vi "rs3 Set All Advanced6.vi"(0 "Set Color Corr":bool=TRUE, 1 "Depth Presets":T2(ring), 2 "Color Presets":T1(ring), 7 "error in (no error)":errorcluster, 8 "device in":u64=370866768, 10 "ST_CensusEnable":cluster{"uDiameter":u32, "vDiameter":u32}={"uDiameter"=9, "vDiameter"=9}, 12 "ST_AE_Control":cluster{"meanIntensitySetpoint":u32}={"meanIntensitySetpoint"=400}, 16 "Depth Table":T3={"depthUnits, um"=1000, "depthClampMin"=0, "depthClampMax"=65535, "disparityMultiplier"=0, "disparityShift"=0}, 17 "ST RAU vector":T9={"minWest"=1, "minEast"=1, "minWEsum"=1, "minNorth"=1, "minSouth"=1, "minNSSum"=1, "uStrink"=1, "vShrink"=1}, 19 "ST Color Control":T8, 20 "depth control":T4={"plusIncrement"=10, "MinusDecrement"=10, "deepSeaMedianThreshold"=528, "scoreThreshA"=10, "scoreThreshB"=1023, "textureDifferenceThreshold"=0, "textureCountThreshold"=0, "deepSeaSecondPeakThreshold"=27, "deepSeaNeighborThreshold"=20, "IrAgreeThreshold"=70}, 21 "STColorCorrection":T11={"colorCorrection 1"=0.54785156, "colorCorrection 2"=0.32910156, "colorCorrection 3"=0.8222656, "colorCorrection 4"=0.109375, "colorCorrection 5"=-0.40527344, "colorCorrection 6"=-1.5253906, "colorCorrection 7"=0.95703125, "colorCorrection 8"=0.89160156, "colorCorrection 9"=0.7675781, "colorCorrection 10"=-0.4794922, "colorCorrection 11"=0.047851562, "colorCorrection 12"=-0.2705078}, 22 "HDAD":T12={"lambdaCensus"=26.0, "lambdaAD"=2100.0, "ignoreSAD"=0}, 23 "ST RSM":T10={"rsmBypass"=0, "diffThresh"=7.0, "sloRauDiffThresh"=3.0, "removeThresh"=33}, 24 "ST SLO Penalty":T5={"sloK1Penalty"=44, "sloK2Penalty"=502, "sloK1PenaltyMod1"=23, "sloK2PenaltyMod1"=237, "sloK1PenaltyMod2"=219, "sloK2PenaltyMod2"=113}, 25 "ST SLO Threshold":T6={"SLOdiffThresholdRed"=300, "SLODiffThresholdGreen"=300, "SLODiffThresholdBlue"=300}, 26 "ST Rau Threshold":T7={"rauDiffThresholdRed"=600, "rauDiffThresholdGreen"=600, "rauDiffThresholdBlue"=600}) -> (14 "Set advanced error":string, 18 "Dev out":u64=370866768, 27 "error out":errorcluster)   [LabVIEW 2019, in "libRealSense3.lvlib"]
doc: "The RealSense D4xx cameras are based on a stereo algorithm that has been accelerated as a fixed-function inside an ASIC. There are many parameters that affect the calculation of the depth. The basic task is to solve the correspondance problem - i.e. figure out which patches in the left image match up to those in the right image by doing a search along an epipolar line (x-axis). The x-axis difference for each object point is known as the disparity. \n\nIn general depth can be estimated for most points in the scene, but some points will have a very low confidence because 1. they are may be occluded (not seen by both imagers), or 2. have very little texture on them which will lead to an ambiquity (ex. when looking at a completely uniform white wall it, there are no best correspondances).\n\nThis VI allows you to set the many parameters that affect the algorith, as well as the color reproduction. \nNote that the color correction matrix will NOT have any effect on the depth calculations."
uses:
  libRealSense3.lvlib
panel:
  # "RS3 Set All Advanced 6"
  # "(C) 2017 Intel Corp.,  AGJ"
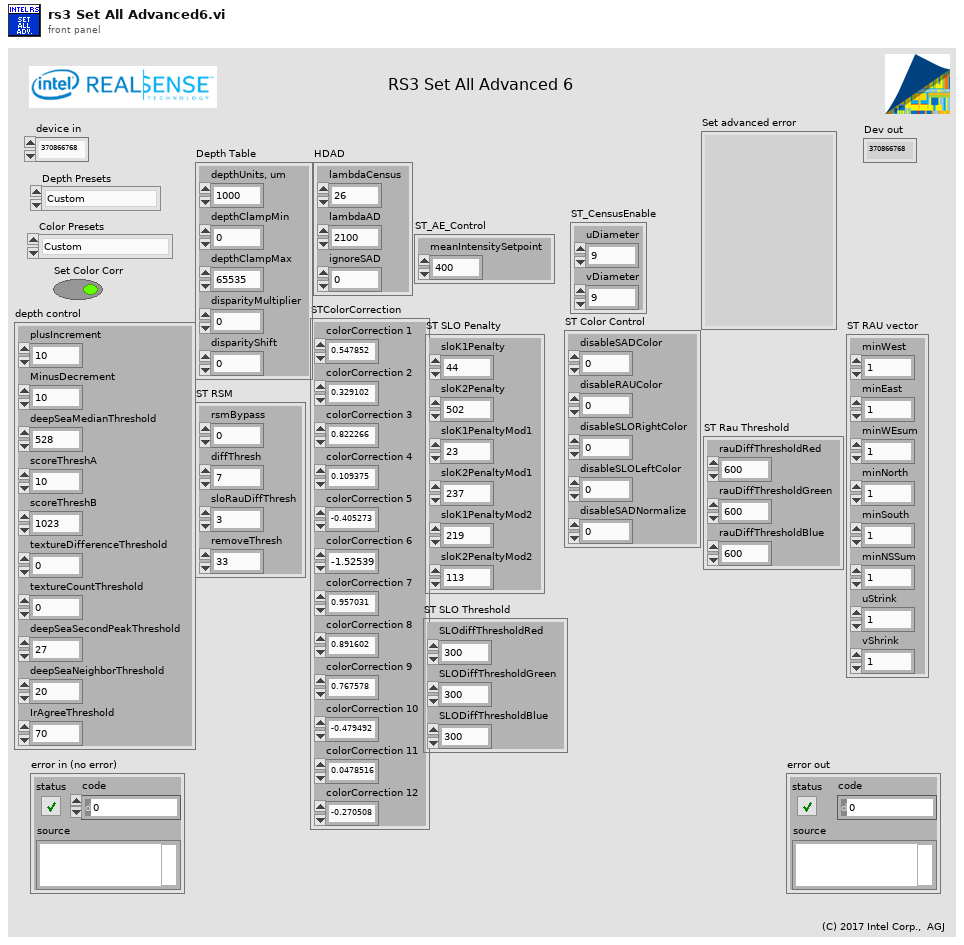
[diagram p1: front panel]
types:
  T1 = enum16{"Custom", "RS400 (DS5p)", "RS400 (DS5p) 2", "RS400 (DS5p) 3", "RS400 (DS5p) 4", "RS400 (DS5p) 5", "RS410 (DS5a)", "RS410 (DS5a) 2", "DS410 (DS5a) 3", "DS410 (DS5a) 4", "DS410+IR", "DS5LR", "DS5LR-2", "DS5LR no pattern", "RS410 Remove IR", "RS410 Remove IR 2", "DS5micro", "D435"}
  T2 = enum16{"Custom", "Original", "New Depth 1", "New Depth 2", "Depth Active 1", "Active 3D Scan", "Active Short A", "Active Short C", "Face", "Face2", "Best Box", "High Density", "Medium Density", "High Accuracy", "Hand", "Short Range", "Flat wall", "Load .JSON", "Load .JSON2"}
  T3 = cluster{"depthUnits, um":u32, "depthClampMin":u32, "depthClampMax":u32, "disparityMultiplier":u32, "disparityShift":u32}
  T4 = cluster{"plusIncrement":u32, "MinusDecrement":u32, "deepSeaMedianThreshold":u32, "scoreThreshA":u32, "scoreThreshB":u32, "textureDifferenceThreshold":u32, "textureCountThreshold":u32, "deepSeaSecondPeakThreshold":u32, "deepSeaNeighborThreshold":u32, "IrAgreeThreshold":u32}
  T5 = cluster{"sloK1Penalty":u32, "sloK2Penalty":u32, "sloK1PenaltyMod1":u32, "sloK2PenaltyMod1":u32, "sloK1PenaltyMod2":u32, "sloK2PenaltyMod2":u32}
  T6 = cluster{"SLOdiffThresholdRed":u32, "SLODiffThresholdGreen":u32, "SLODiffThresholdBlue":u32}
  T7 = cluster{"rauDiffThresholdRed":u32, "rauDiffThresholdGreen":u32, "rauDiffThresholdBlue":u32}
  T8 = cluster{"disableSADColor":u32, "disableRAUColor":u32, "disableSLORightColor":u32, "disableSLOLeftColor":u32, "disableSADNormalize":u32}
  T9 = cluster{"minWest":u32, "minEast":u32, "minWEsum":u32, "minNorth":u32, "minSouth":u32, "minNSSum":u32, "uStrink":u32, "vShrink":u32}
  T10 = cluster{"rsmBypass":u32, "diffThresh":sgl, "sloRauDiffThresh":sgl, "removeThresh":u32}
  T11 = cluster{"colorCorrection 1":sgl, "colorCorrection 2":sgl, "colorCorrection 3":sgl, "colorCorrection 4":sgl, "colorCorrection 5":sgl, "colorCorrection 6":sgl, "colorCorrection 7":sgl, "colorCorrection 8":sgl, "colorCorrection 9":sgl, "colorCorrection 10":sgl, "colorCorrection 11":sgl, "colorCorrection 12":sgl}
  T12 = cluster{"lambdaCensus":sgl, "lambdaAD":sgl, "ignoreSAD":u32}
  T13 = cluster{"rsmBypass (56)":u32, "diffThresh (57)":sgl, "sloRauDiffThresh(58)":sgl, "removeThresh(59)":u32}
  T14 = cluster{"depth control":cluster{"plusIncrement":u32, "MinusDecrement":u32, "deepSeaMedianThreshold":u32, "scoreThreshA":u32, "scoreThreshB":u32, "textureDifferenceThreshold":u32, "textureCountThreshold":u32, "deepSeaSecondPeakThreshold":u32, "deepSeaNeighborThreshold":u32, "IrAgreeThreshold":u32}, "STColorCorrection output":cluster{"colorCorrection 1":sgl, "colorCorrection 2":sgl, "colorCorrection 3":sgl, "colorCorrection 4":sgl, "colorCorrection 5":sgl, "colorCorrection 6":sgl, "colorCorrection 7":sgl, "colorCorrection 8":sgl, "colorCorrection 9":sgl, "colorCorrection 10":sgl, "colorCorrection 11":sgl, "colorCorrection 12":sgl}, "HDAD":cluster{"lambdaCensus":sgl, "lambdaAD":sgl, "ignoreSAD":u32}, "ST RSM":cluster{"rsmBypass":u32, "diffThresh":sgl, "sloRauDiffThresh":sgl, "removeThresh":u32}, "ST SLO Penalty":cluster{"sloK1Penalty":u32, "sloK2Penalty":u32, "sloK1PenaltyMod1":u32, "sloK2PenaltyMod1":u32, "sloK1PenaltyMod2":u32, "sloK2PenaltyMod2":u32}, "ST SLO Threshold":cluster{"SLOdiffThresholdRed":u32, "SLODiffThresholdGreen":u32, "SLODiffThresholdBlue":u32}, "ST Rau Threshold":cluster{"rauDiffThresholdRed":u32, "rauDiffThresholdGreen":u32, "rauDiffThresholdBlue":u32}, "ST Color Control":cluster{"disableSADColor":u32, "disableRAUColor":u32, "disableSLORightColor":u32, "disableSLOLeftColor":u32, "disableSADNormalize":u32}, "ST RAU vector":cluster{"minWest":u32, "minEast":u32, "minWEsum":u32, "minNorth":u32, "minSouth":u32, "minNSSum":u32, "uStrink":u32, "vShrink":u32}, "Depth Table":cluster{"depthUnits, um":u32, "depthClampMin":u32, "depthClampMax":u32, "disparityMultiplier":u32, "disparityShift":u32}, "ST_AE_Control":cluster{"meanIntensitySetpoint":u32}, "ST_CensusEnable":cluster{"uDiameter":u32, "vDiameter":u32}}
  T15 = cluster{"depthUnits, um":u32, "depthClampMin":u32, "depthClampMax":u32, "disparityMultiplier":u32, "disparityShift(0-127)":u32}
  T16 = cluster{"minWest (60)":u32, "minEast (61)":u32, "minWEsum (62)":u32, "minNorth (63)":u32, "minSouth (64)":u32, "minNSSum(65)":u32, "uStrink (66)":u32, "vShrink (67)":u32}
  T17 = cluster{"rauDiffThreshRed(73)":u32, "rauDiffThreshGreen(74)":u32, "rauDiffThreshBlue(75)":u32}
  T18 = cluster{"sloK1Penalty (79)":u32, "sloK2Penalty (80)":u32, "sloK1PenaltyMod1(81)":u32, "sloK2PenaltyMod1(82)":u32, "sloK1PenaltyMod2(83)":u32, "sloK2PenaltyMod2(84)":u32}
  T19 = cluster{"SLOdiffThreshRed(76)":u32, "SLODiffThreshGreen(77)":u32, "SLODiffThreshBlue(78)":u32}
  T20 = cluster{"disableSADColor(68)":u32, "disableRAUColor(69)":u32, "disableSLORightColor(70)":u32, "disableSLOLeftColor(71)":u32, "disableSADNormalize(72)":u32}
  T21 = cluster{"plusIncrement (47)":u32, "MinusDecrement (46)":u32, "deepSeaMedianThreshold (48)":u32, "scoreThreshA(49)":u32, "scoreThreshB (50)":u32, "textureDifferenceThreshold (52)":u32, "textureCountThreshold (51)":u32, "deepSea2ndPeakThresh.(53)":u32, "deepSeaNeighborThresh.(54)":u32, "LRAgreeThreshold (55)":u32}
  T22 = cluster{"plusIncrement (47)":u32, "MinusDecrement (46)":u32, "deepSeaMedianThreshold (48)":u32, "scoreThreshA(49)":u32, "scoreThreshB (50)":u32, "textureDifferenceThreshold (52)":u32, "textureCountThreshold (51)":u32, "deepSea2ndPeakThresh.(53)":u32, "deepSeaNeighborThresh.(54)":u32, "IrAgreeThreshold (55)":u32}
  T23 = cluster{"DS5p- 1":sgl, "colorCorrection 2":sgl, "colorCorrection 3":sgl, "colorCorrection 4":sgl, "colorCorrection 5":sgl, "colorCorrection 6":sgl, "colorCorrection 7":sgl, "colorCorrection 8":sgl, "colorCorrection 9":sgl, "colorCorrection 10":sgl, "colorCorrection 11":sgl, "colorCorrection 12":sgl}
  T24 = cluster{"Color 0":dbl, "Color 1":dbl, "Color 2":dbl, "Color 3":dbl, "Color 4":dbl, "Color 5":dbl, "Color 6":dbl, "Color 7":dbl, "Color 8":dbl, "Color 9":dbl, "Color 10":dbl, "Color 11":dbl}
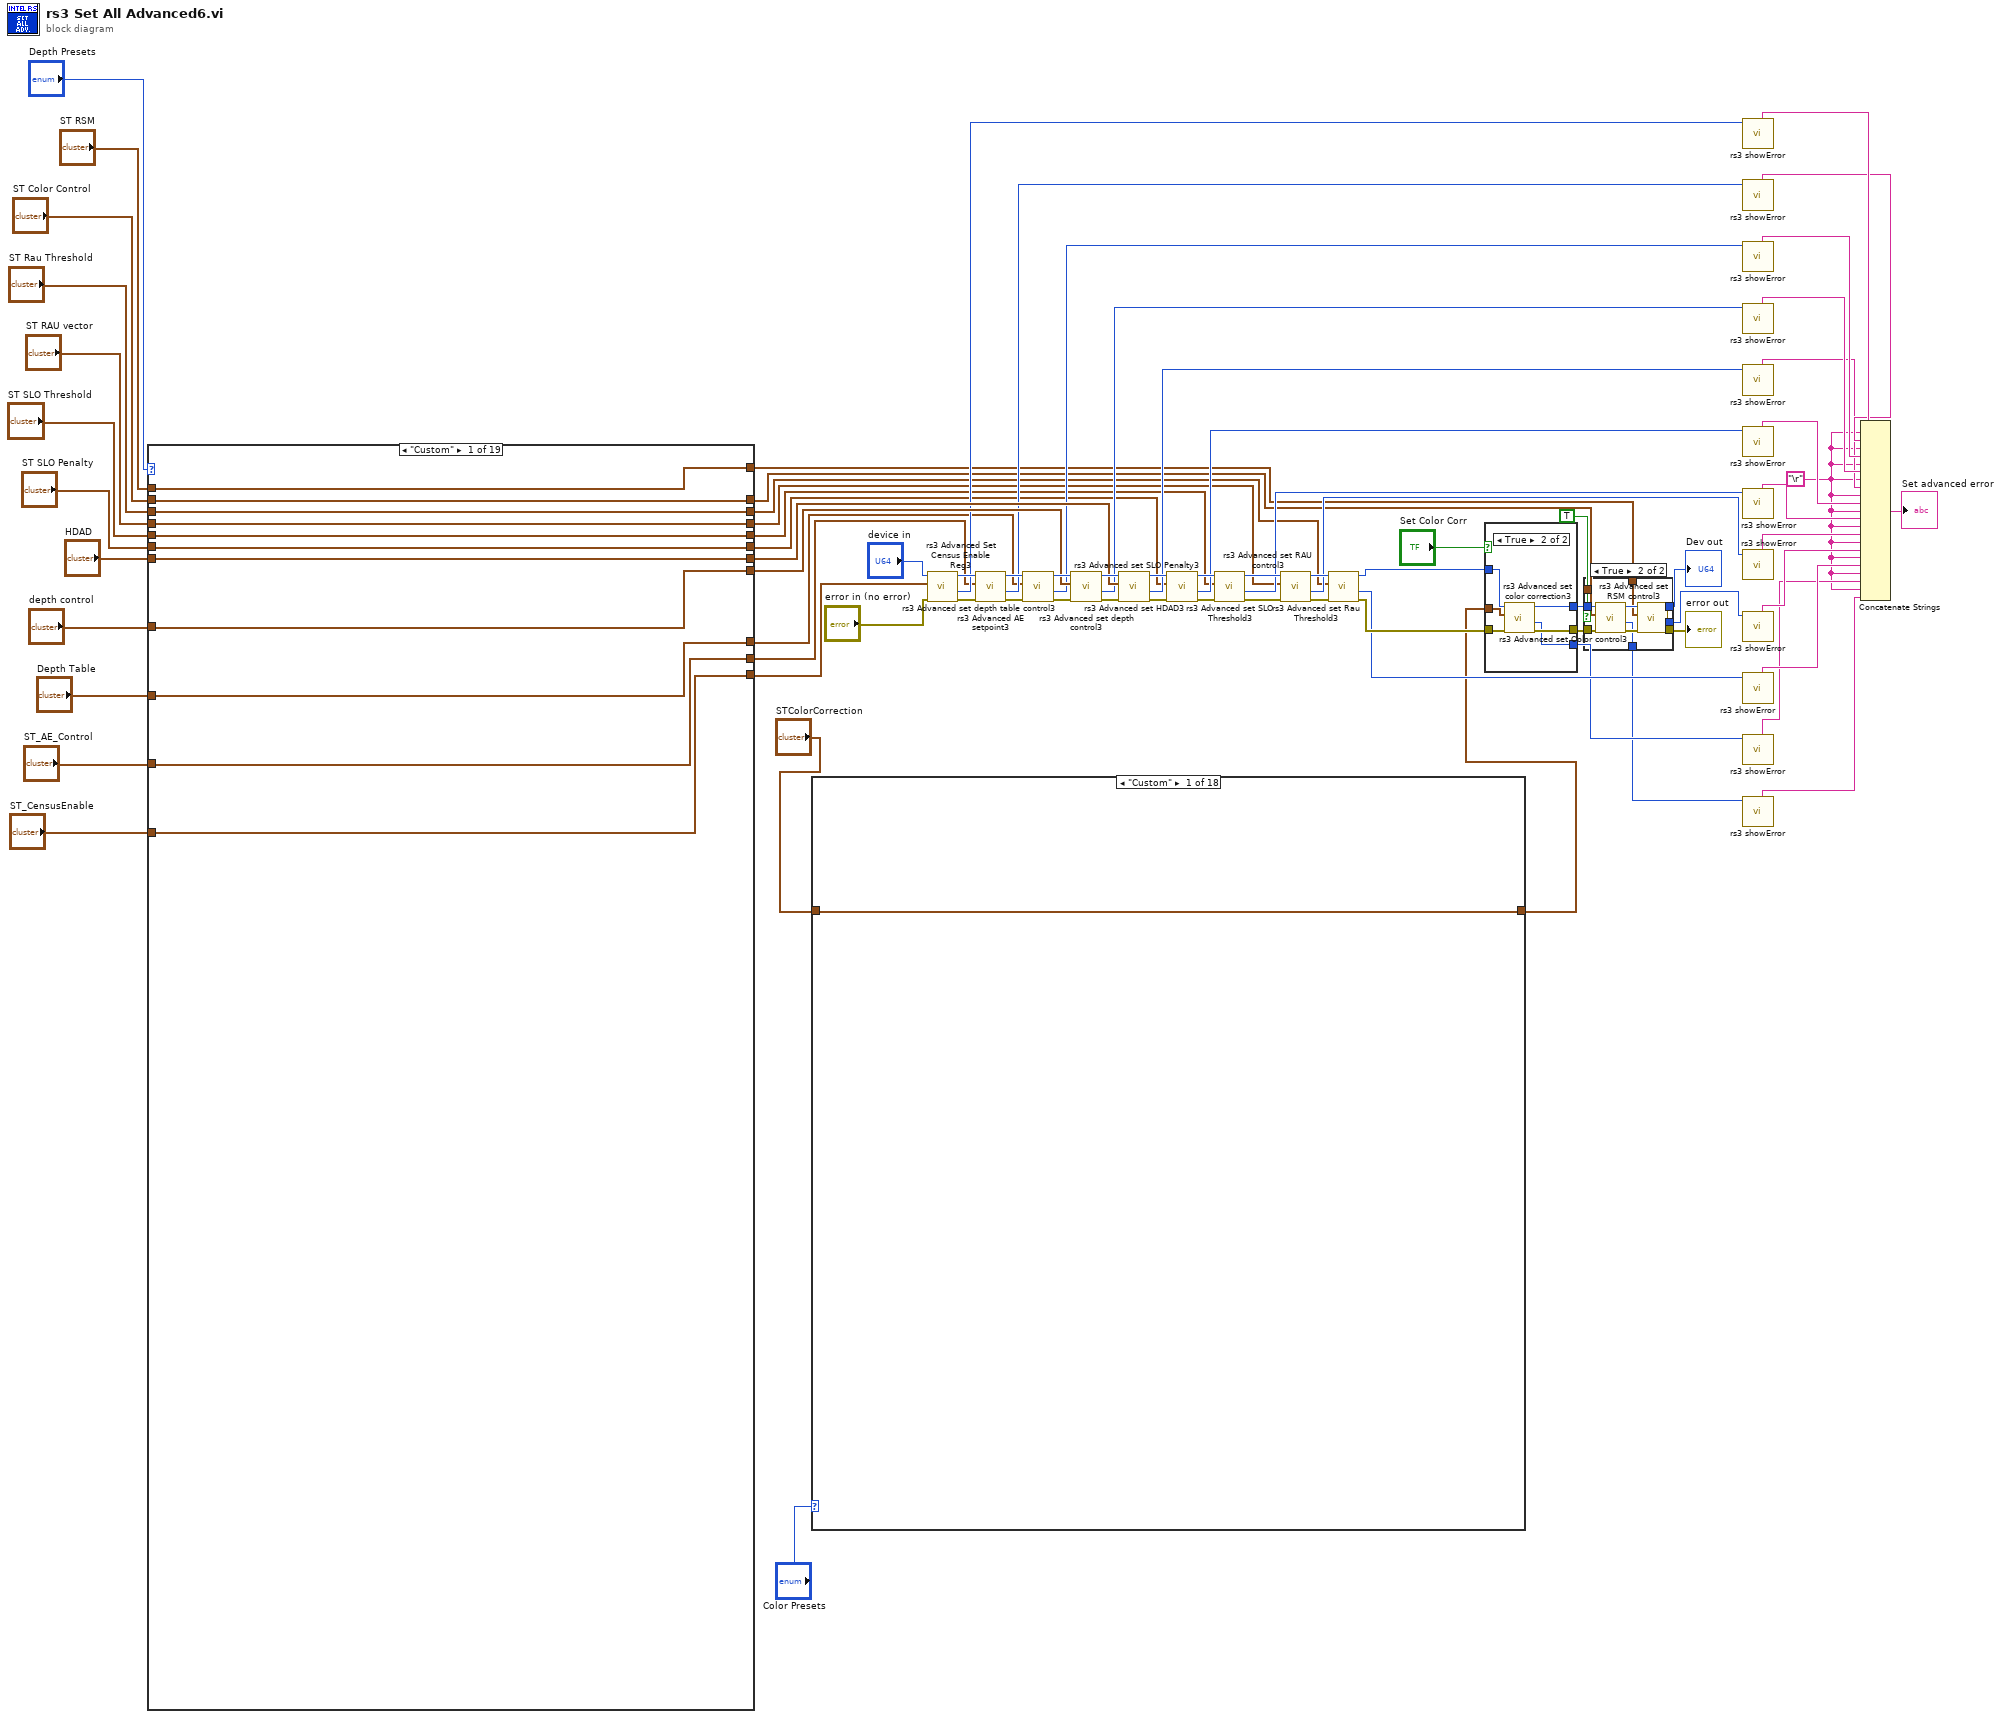
[diagram p0: block diagram]
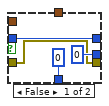
[diagram p2: hidden frame]
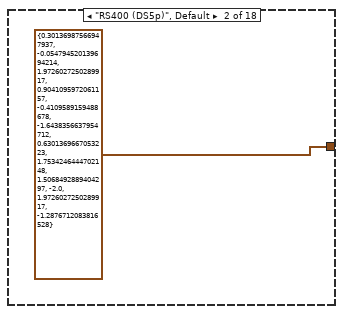
[diagram p3: hidden frame]
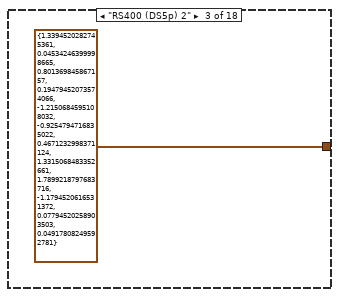
[diagram p4: hidden frame]
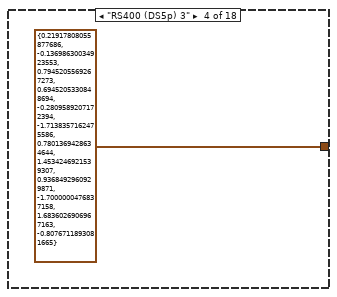
[diagram p5: hidden frame]
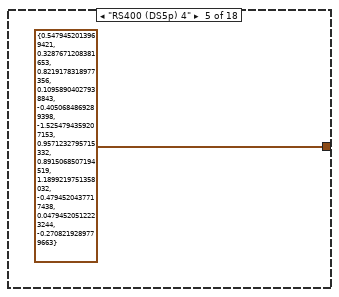
[diagram p6: hidden frame]
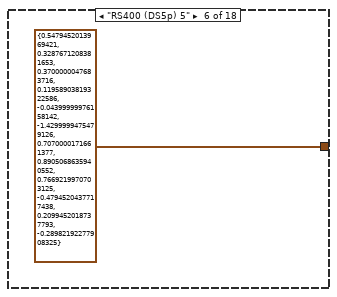
[diagram p7: hidden frame]
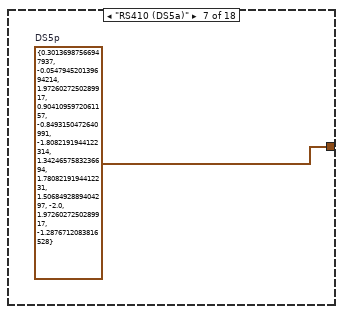
[diagram p8: hidden frame]
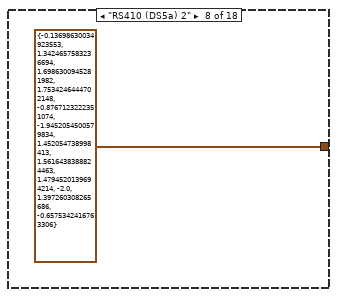
[diagram p9: hidden frame]
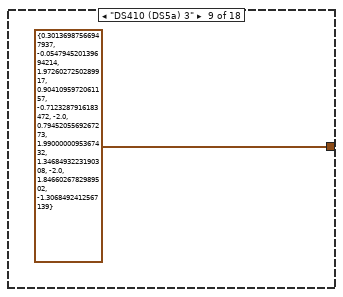
[diagram p10: hidden frame]
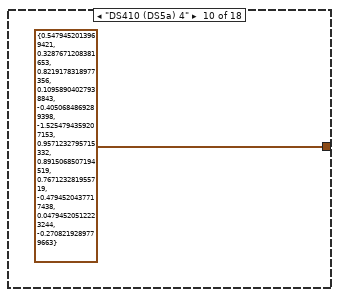
[diagram p11: hidden frame]
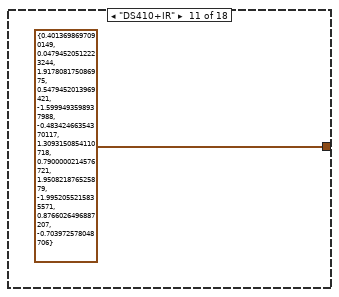
[diagram p12: hidden frame]
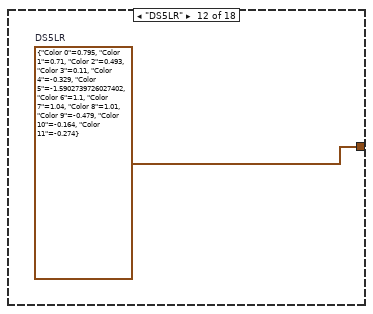
[diagram p13: hidden frame]
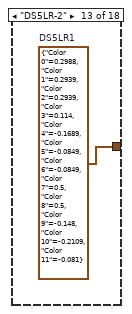
[diagram p14: hidden frame]
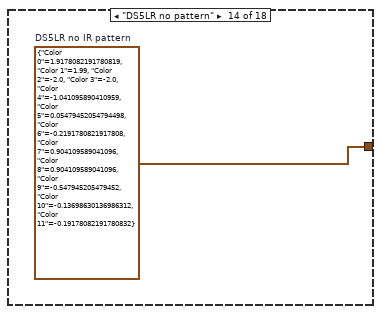
[diagram p15: hidden frame]
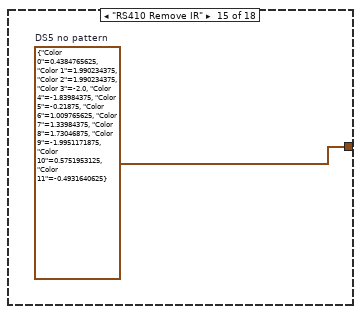
[diagram p16: hidden frame]
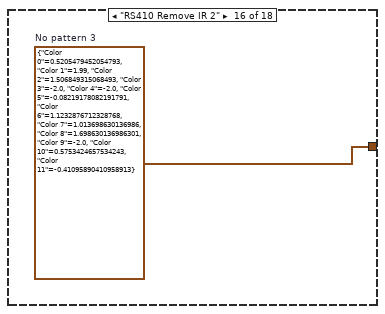
[diagram p17: hidden frame]
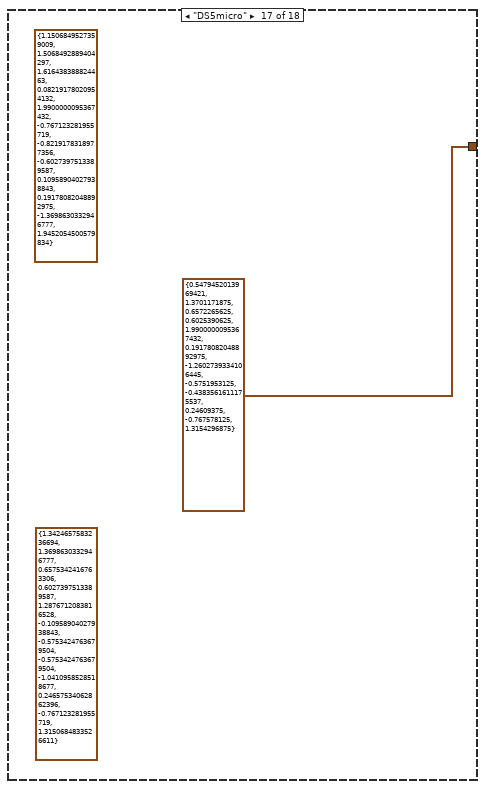
[diagram p18: hidden frame]
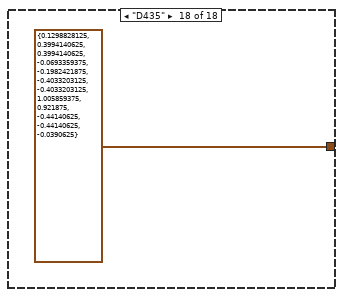
[diagram p19: hidden frame]
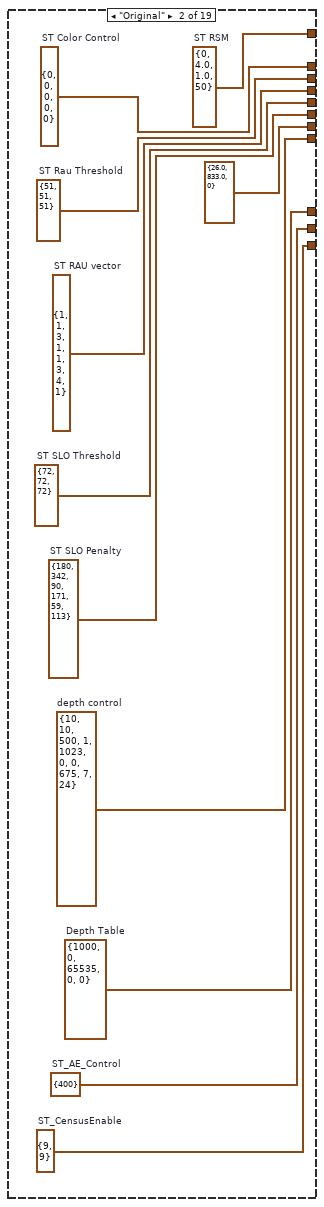
[diagram p20: hidden frame]
diagram:
  w24 = "\r"
  n1 = case shown="\"Custom\"" "Depth Presets" {
    tunnel: [w89 w99 w111 w122 w133 w137 w148 w159 w175 w185 w196 w203 w216 w228 w240 w252 w264 w279 w293] -> w51
    tunnel: [w83 w98 w110 w121 w132 T13 {"rsmBypass (56)"=0, "diffThresh (57)"=1.0367311, "sloRauDiffThresh(58)"=151.0, "removeThresh(59)"=1} ("ST RSM 2") w155 w166 w177 w182 w193 w208 w221 w233 w245 w257 w269 w281 w295] -> w13
    tunnel: [w84 w93 w109 w120 w131 w144 w154 w165 w176 w183 w194 w210 w223 w235 w247 w259 w271 w278 w292] -> w15
    tunnel: [w85 w94 w108 w119 w130 w143 w153 w164 w173 w184 w195 w206 w219 w231 w243 w255 w267 w282 w296] -> w16
    tunnel: [w82 w97 w107 w118 w129 w142 w152 w163 w172 w186 w197 w202 w215 w227 w239 w251 w263 w285 w299] -> w11
    tunnel: [w86 w96 w106 w117 w128 w141 w151 w162 w170 w187 w198 w201 w214 w226 w238 w250 w262 w284 w298] -> w18
    tunnel: [w87 w95 w105 w116 w127 w140 w150 w161 w174 w188 w199 w200 w213 w225 w237 w249 w261 w283 w297] -> w21
    tunnel: [w88 T12 {"lambdaCensus"=26.0, "lambdaAD"=833.0, "ignoreSAD"=0} ("HDAD 2") T12 {"lambdaCensus"=126.0, "lambdaAD"=800.0, "ignoreSAD"=0} ("HDAD 2") T12 {"lambdaCensus"=200.0, "lambdaAD"=1900.0, "ignoreSAD"=0} ("HDAD 2") T12 {"lambdaCensus"=216.0, "lambdaAD"=1400.0, "ignoreSAD"=0} ("HDAD 2") T12 {"lambdaCensus"=26.0, "lambdaAD"=833.0, "ignoreSAD"=0} ("HDAD 2") T12 {"lambdaCensus"=100.0, "lambdaAD"=1600.0, "ignoreSAD"=0} ("HDAD 2") w160 w171 T12 {"lambdaCensus"=26.0, "lambdaAD"=2100.0, "ignoreSAD"=0} ("HDAD*") T12 {"lambdaCensus"=15.0, "lambdaAD"=618.0, "ignoreSAD"=0} ("HDAD*") w209 w222 w234 w246 w258 w270 w280 w294] -> w49
    tunnel: [w80 w90 w101 w112 w123 w134 w145 w157 w167 w178 w189 w204 w217 w229 w241 w253 w265 w272 w288] -> w7
    tunnel: [w81 w91 w102 w113 w124 w135 w146 w156 w168 w179 w190 w205 w218 w230 w242 w254 w266 w273 w287] -> w9
    tunnel: [w79 w92 w103 w114 w125 w136 w147 w158 w169 w180 w191 w207 w220 w232 w244 w256 w268 w274 w286] -> w5
    tunnel: "depth control" -> [w89 _ _ _ _ _ _ _ _ _ _ _ _ _ _ _ _ _ _]
    tunnel: "HDAD" -> [w88 _ _ _ _ _ _ _ _ _ _ _ _ _ _ _ _ _ _]
    tunnel: "ST SLO Penalty" -> [w87 _ _ _ _ _ _ _ _ _ _ _ _ _ _ _ _ _ _]
    tunnel: "ST SLO Threshold" -> [w86 _ _ _ _ _ _ _ _ _ _ _ _ _ _ _ _ _ _]
    tunnel: "ST RAU vector" -> [w84 _ _ _ _ _ _ _ _ _ _ _ _ _ _ _ _ _ _]
    tunnel: "ST Rau Threshold" -> [w85 _ _ _ _ _ _ _ _ _ _ _ _ _ _ _ _ _ _]
    tunnel: "ST RSM" -> [w83 _ _ _ _ _ _ _ _ _ _ _ _ _ _ _ _ _ _]
    tunnel: "ST Color Control" -> [w82 _ _ _ _ _ _ _ _ _ _ _ _ _ _ _ _ _ _]
    tunnel: "ST_CensusEnable" -> [w81 _ _ _ _ _ _ _ _ _ _ _ _ _ _ _ _ _ _]
    tunnel: "ST_AE_Control" -> [w80 _ _ _ _ _ _ _ _ _ _ _ _ _ _ _ _ _ _]
    tunnel: "Depth Table" -> [w79 _ _ _ _ _ _ _ _ _ _ _ _ _ _ _ _ _ _]
    frame "Custom" {
    }
    frame "Original" {
      w91 = cluster{"uDiameter":u32, "vDiameter":u32} {"uDiameter"=9, "vDiameter"=9}  # ST_CensusEnable
      w92 = T15 {"depthUnits, um"=1000, "depthClampMin"=0, "depthClampMax"=65535, "disparityMultiplier"=0, "disparityShift(0-127)"=0}  # Depth Table
      w90 = cluster{"meanIntensitySetpoint":u32} {"meanIntensitySetpoint"=400}  # ST_AE_Control
      w93 = T16 {"minWest (60)"=1, "minEast (61)"=1, "minWEsum (62)"=3, "minNorth (63)"=1, "minSouth (64)"=1, "minNSSum(65)"=3, "uStrink (66)"=4, "vShrink (67)"=1}  # ST RAU vector
      w94 = T17 {"rauDiffThreshRed(73)"=51, "rauDiffThreshGreen(74)"=51, "rauDiffThreshBlue(75)"=51}  # ST Rau Threshold
      w95 = T18 {"sloK1Penalty (79)"=180, "sloK2Penalty (80)"=342, "sloK1PenaltyMod1(81)"=90, "sloK2PenaltyMod1(82)"=171, "sloK1PenaltyMod2(83)"=59, "sloK2PenaltyMod2(84)"=113}  # ST SLO Penalty
      w96 = T19 {"SLOdiffThreshRed(76)"=72, "SLODiffThreshGreen(77)"=72, "SLODiffThreshBlue(78)"=72}  # ST SLO Threshold
      w97 = T20 {"disableSADColor(68)"=0, "disableRAUColor(69)"=0, "disableSLORightColor(70)"=0, "disableSLOLeftColor(71)"=0, "disableSADNormalize(72)"=0}  # ST Color Control
      w98 = T13 {"rsmBypass (56)"=0, "diffThresh (57)"=4.0, "sloRauDiffThresh(58)"=1.0, "removeThresh(59)"=50}  # ST RSM
      w99 = T21 {"plusIncrement (47)"=10, "MinusDecrement (46)"=10, "deepSeaMedianThreshold (48)"=500, "scoreThreshA(49)"=1, "scoreThreshB (50)"=1023, "textureDifferenceThreshold (52)"=0, "textureCountThreshold (51)"=0, "deepSea2ndPeakThresh.(53)"=675, "deepSeaNeighborThresh.(54)"=7, "LRAgreeThreshold (55)"=24}  # depth control
    }
    frame "New Depth 1", Default {
      w102 = cluster{"uDiameter":u32, "vDiameter":u32} {"uDiameter"=9, "vDiameter"=9}  # ST_CensusEnable
      w103 = T15 {"depthUnits, um"=1000, "depthClampMin"=0, "depthClampMax"=65535, "disparityMultiplier"=0, "disparityShift(0-127)"=0}  # Depth Table
      w101 = cluster{"meanIntensitySetpoint":u32} {"meanIntensitySetpoint"=400}  # ST_AE_Control
      w105 = T18 {"sloK1Penalty (79)"=42, "sloK2Penalty (80)"=191, "sloK1PenaltyMod1(81)"=84, "sloK2PenaltyMod1(82)"=4, "sloK1PenaltyMod2(83)"=59, "sloK2PenaltyMod2(84)"=4}  # ST SLO Penalty 2
      w106 = T19 {"SLOdiffThreshRed(76)"=43, "SLODiffThreshGreen(77)"=83, "SLODiffThreshBlue(78)"=72}  # ST SLO Threshold 2
      w107 = T20 {"disableSADColor(68)"=0, "disableRAUColor(69)"=0, "disableSLORightColor(70)"=0, "disableSLOLeftColor(71)"=0, "disableSADNormalize(72)"=0}  # ST Color Control 2
      w108 = T17 {"rauDiffThreshRed(73)"=1, "rauDiffThreshGreen(74)"=1, "rauDiffThreshBlue(75)"=1}  # ST Rau Threshold 2
      w109 = T16 {"minWest (60)"=7, "minEast (61)"=7, "minWEsum (62)"=12, "minNorth (63)"=3, "minSouth (64)"=2, "minNSSum(65)"=1, "uStrink (66)"=2, "vShrink (67)"=1}  # ST RAU vector 2
      w110 = T13 {"rsmBypass (56)"=0, "diffThresh (57)"=6.49, "sloRauDiffThresh(58)"=0.305, "removeThresh(59)"=70}  # ST RSM 2
      w111 = T22 {"plusIncrement (47)"=4, "MinusDecrement (46)"=1, "deepSeaMedianThreshold (48)"=95, "scoreThreshA(49)"=13, "scoreThreshB (50)"=1023, "textureDifferenceThreshold (52)"=499, "textureCountThreshold (51)"=0, "deepSea2ndPeakThresh.(53)"=1, "deepSeaNeighborThresh.(54)"=5, "IrAgreeThreshold (55)"=32}  # depth control 2
    }
    frame "New Depth 2" {
      w113 = cluster{"uDiameter":u32, "vDiameter":u32} {"uDiameter"=9, "vDiameter"=9}  # ST_CensusEnable
      w114 = T15 {"depthUnits, um"=1000, "depthClampMin"=0, "depthClampMax"=65535, "disparityMultiplier"=0, "disparityShift(0-127)"=0}  # Depth Table
      w112 = cluster{"meanIntensitySetpoint":u32} {"meanIntensitySetpoint"=400}  # ST_AE_Control
      w116 = T18 {"sloK1Penalty (79)"=42, "sloK2Penalty (80)"=191, "sloK1PenaltyMod1(81)"=84, "sloK2PenaltyMod1(82)"=4, "sloK1PenaltyMod2(83)"=59, "sloK2PenaltyMod2(84)"=4}  # ST SLO Penalty 2
      w117 = T19 {"SLOdiffThreshRed(76)"=100, "SLODiffThreshGreen(77)"=100, "SLODiffThreshBlue(78)"=100}  # ST SLO Threshold 2
      w118 = T20 {"disableSADColor(68)"=0, "disableRAUColor(69)"=0, "disableSLORightColor(70)"=0, "disableSLOLeftColor(71)"=0, "disableSADNormalize(72)"=0}  # ST Color Control 2
      w119 = T17 {"rauDiffThreshRed(73)"=50, "rauDiffThreshGreen(74)"=50, "rauDiffThreshBlue(75)"=50}  # ST Rau Threshold 2
      w120 = T16 {"minWest (60)"=1, "minEast (61)"=1, "minWEsum (62)"=9, "minNorth (63)"=3, "minSouth (64)"=2, "minNSSum(65)"=1, "uStrink (66)"=2, "vShrink (67)"=1}  # ST RAU vector 2
      w121 = T13 {"rsmBypass (56)"=0, "diffThresh (57)"=6.49, "sloRauDiffThresh(58)"=0.305, "removeThresh(59)"=50}  # ST RSM 2
      w122 = T22 {"plusIncrement (47)"=4, "MinusDecrement (46)"=1, "deepSeaMedianThreshold (48)"=95, "scoreThreshA(49)"=13, "scoreThreshB (50)"=1023, "textureDifferenceThreshold (52)"=499, "textureCountThreshold (51)"=0, "deepSea2ndPeakThresh.(53)"=1, "deepSeaNeighborThresh.(54)"=5, "IrAgreeThreshold (55)"=200}  # depth control 2
    }
    frame "Depth Active 1" {
      w124 = cluster{"uDiameter":u32, "vDiameter":u32} {"uDiameter"=9, "vDiameter"=9}  # ST_CensusEnable
      w125 = T15 {"depthUnits, um"=1000, "depthClampMin"=0, "depthClampMax"=65535, "disparityMultiplier"=0, "disparityShift(0-127)"=0}  # Depth Table
      w123 = cluster{"meanIntensitySetpoint":u32} {"meanIntensitySetpoint"=400}  # ST_AE_Control
      w127 = T18 {"sloK1Penalty (79)"=10, "sloK2Penalty (80)"=60, "sloK1PenaltyMod1(81)"=84, "sloK2PenaltyMod1(82)"=56, "sloK1PenaltyMod2(83)"=59, "sloK2PenaltyMod2(84)"=4}  # ST SLO Penalty 2
      w128 = T19 {"SLOdiffThreshRed(76)"=200, "SLODiffThreshGreen(77)"=200, "SLODiffThreshBlue(78)"=200}  # ST SLO Threshold 2
      w129 = T20 {"disableSADColor(68)"=0, "disableRAUColor(69)"=0, "disableSLORightColor(70)"=0, "disableSLOLeftColor(71)"=0, "disableSADNormalize(72)"=0}  # ST Color Control 2
      w130 = T17 {"rauDiffThreshRed(73)"=70, "rauDiffThreshGreen(74)"=70, "rauDiffThreshBlue(75)"=70}  # ST Rau Threshold 2
      w131 = T16 {"minWest (60)"=7, "minEast (61)"=7, "minWEsum (62)"=12, "minNorth (63)"=3, "minSouth (64)"=2, "minNSSum(65)"=1, "uStrink (66)"=2, "vShrink (67)"=1}  # ST RAU vector 2
      w132 = T13 {"rsmBypass (56)"=0, "diffThresh (57)"=6.49, "sloRauDiffThresh(58)"=0.305, "removeThresh(59)"=60}  # ST RSM 2
      w133 = T22 {"plusIncrement (47)"=4, "MinusDecrement (46)"=1, "deepSeaMedianThreshold (48)"=95, "scoreThreshA(49)"=13, "scoreThreshB (50)"=1023, "textureDifferenceThreshold (52)"=499, "textureCountThreshold (51)"=0, "deepSea2ndPeakThresh.(53)"=1, "deepSeaNeighborThresh.(54)"=5, "IrAgreeThreshold (55)"=82}  # depth control 2
    }
    frame "Active 3D Scan" {
      w135 = cluster{"uDiameter":u32, "vDiameter":u32} {"uDiameter"=9, "vDiameter"=9}  # ST_CensusEnable
      w136 = T15 {"depthUnits, um"=1000, "depthClampMin"=0, "depthClampMax"=65535, "disparityMultiplier"=0, "disparityShift(0-127)"=0}  # Depth Table
      w134 = cluster{"meanIntensitySetpoint":u32} {"meanIntensitySetpoint"=400}  # ST_AE_Control
      w137 = T22 {"plusIncrement (47)"=19, "MinusDecrement (46)"=4, "deepSeaMedianThreshold (48)"=554, "scoreThreshA(49)"=1, "scoreThreshB (50)"=632, "textureDifferenceThreshold (52)"=0, "textureCountThreshold (51)"=31, "deepSea2ndPeakThresh.(53)"=665, "deepSeaNeighborThresh.(54)"=126, "IrAgreeThreshold (55)"=11}  # depth control 2
      w140 = T18 {"sloK1Penalty (79)"=93, "sloK2Penalty (80)"=473, "sloK1PenaltyMod1(81)"=70, "sloK2PenaltyMod1(82)"=123, "sloK1PenaltyMod2(83)"=92, "sloK2PenaltyMod2(84)"=409}  # ST SLO Penalty 2
      w141 = T19 {"SLOdiffThreshRed(76)"=46, "SLODiffThreshGreen(77)"=442, "SLODiffThreshBlue(78)"=105}  # ST SLO Threshold 2
      w142 = T20 {"disableSADColor(68)"=0, "disableRAUColor(69)"=0, "disableSLORightColor(70)"=0, "disableSLOLeftColor(71)"=0, "disableSADNormalize(72)"=0}  # ST Color Control 2
      w143 = T17 {"rauDiffThreshRed(73)"=46, "rauDiffThreshGreen(74)"=442, "rauDiffThreshBlue(75)"=105}  # ST Rau Threshold 2
      w144 = T16 {"minWest (60)"=5, "minEast (61)"=7, "minWEsum (62)"=12, "minNorth (63)"=1, "minSouth (64)"=3, "minNSSum(65)"=7, "uStrink (66)"=4, "vShrink (67)"=1}  # ST RAU vector 2
    }
    frame "Active Short A" {
      w146 = cluster{"uDiameter":u32, "vDiameter":u32} {"uDiameter"=3, "vDiameter"=3}  # ST_CensusEnable
      w147 = T15 {"depthUnits, um"=200, "depthClampMin"=0, "depthClampMax"=65535, "disparityMultiplier"=0, "disparityShift(0-127)"=0}  # Depth Table
      w145 = cluster{"meanIntensitySetpoint":u32} {"meanIntensitySetpoint"=400}  # ST_AE_Control
      w148 = T22 {"plusIncrement (47)"=7, "MinusDecrement (46)"=1, "deepSeaMedianThreshold (48)"=140, "scoreThreshA(49)"=10, "scoreThreshB (50)"=1023, "textureDifferenceThreshold (52)"=499, "textureCountThreshold (51)"=0, "deepSea2ndPeakThresh.(53)"=1, "deepSeaNeighborThresh.(54)"=5, "IrAgreeThreshold (55)"=80}  # depth control 2
      w150 = T18 {"sloK1Penalty (79)"=5, "sloK2Penalty (80)"=30, "sloK1PenaltyMod1(81)"=11, "sloK2PenaltyMod1(82)"=50, "sloK1PenaltyMod2(83)"=56, "sloK2PenaltyMod2(84)"=15}  # ST SLO Penalty 2
      w151 = T19 {"SLOdiffThreshRed(76)"=200, "SLODiffThreshGreen(77)"=200, "SLODiffThreshBlue(78)"=200}  # ST SLO Threshold 2
      w152 = T20 {"disableSADColor(68)"=0, "disableRAUColor(69)"=0, "disableSLORightColor(70)"=0, "disableSLOLeftColor(71)"=0, "disableSADNormalize(72)"=0}  # ST Color Control 2
      w153 = T17 {"rauDiffThreshRed(73)"=200, "rauDiffThreshGreen(74)"=200, "rauDiffThreshBlue(75)"=200}  # ST Rau Threshold 2
      w154 = T16 {"minWest (60)"=3, "minEast (61)"=3, "minWEsum (62)"=13, "minNorth (63)"=1, "minSouth (64)"=1, "minNSSum(65)"=1, "uStrink (66)"=4, "vShrink (67)"=4}  # ST RAU vector 2
      w155 = T13 {"rsmBypass (56)"=0, "diffThresh (57)"=7.5, "sloRauDiffThresh(58)"=0.9, "removeThresh(59)"=72}  # ST RSM 2
    }
    frame "Active Short C" {
      w156 = cluster{"uDiameter":u32, "vDiameter":u32} {"uDiameter"=3, "vDiameter"=3}  # ST_CensusEnable
      w158 = T15 {"depthUnits, um"=200, "depthClampMin"=0, "depthClampMax"=65535, "disparityMultiplier"=0, "disparityShift(0-127)"=0}  # Depth Table
      w157 = cluster{"meanIntensitySetpoint":u32} {"meanIntensitySetpoint"=400}  # ST_AE_Control
      w159 = T22 {"plusIncrement (47)"=10, "MinusDecrement (46)"=10, "deepSeaMedianThreshold (48)"=415, "scoreThreshA(49)"=1, "scoreThreshB (50)"=1023, "textureDifferenceThreshold (52)"=0, "textureCountThreshold (51)"=14, "deepSea2ndPeakThresh.(53)"=56, "deepSeaNeighborThresh.(54)"=108, "IrAgreeThreshold (55)"=8}  # depth control 2
      w160 = T12 {"lambdaCensus"=26.0, "lambdaAD"=958.0, "ignoreSAD"=0}  # HDAD 2
      w161 = T18 {"sloK1Penalty (79)"=203, "sloK2Penalty (80)"=342, "sloK1PenaltyMod1(81)"=109, "sloK2PenaltyMod1(82)"=502, "sloK1PenaltyMod2(83)"=209, "sloK2PenaltyMod2(84)"=14}  # ST SLO Penalty 2
      w162 = T19 {"SLOdiffThreshRed(76)"=889, "SLODiffThreshGreen(77)"=69, "SLODiffThreshBlue(78)"=189}  # ST SLO Threshold 2
      w163 = T20 {"disableSADColor(68)"=0, "disableRAUColor(69)"=0, "disableSLORightColor(70)"=0, "disableSLOLeftColor(71)"=0, "disableSADNormalize(72)"=0}  # ST Color Control 2
      w164 = T17 {"rauDiffThreshRed(73)"=298, "rauDiffThreshGreen(74)"=95, "rauDiffThreshBlue(75)"=675}  # ST Rau Threshold 2
      w165 = T16 {"minWest (60)"=1, "minEast (61)"=1, "minWEsum (62)"=3, "minNorth (63)"=1, "minSouth (64)"=1, "minNSSum(65)"=3, "uStrink (66)"=3, "vShrink (67)"=1}  # ST RAU vector 2
      w166 = T13 {"rsmBypass (56)"=0, "diffThresh (57)"=5.386, "sloRauDiffThresh(58)"=0.9687, "removeThresh(59)"=88}  # ST RSM 2
    }
    frame "Face" {
      w168 = cluster{"uDiameter":u32, "vDiameter":u32} {"uDiameter"=9, "vDiameter"=9}  # ST_CensusEnable
      w169 = T15 {"depthUnits, um"=1000, "depthClampMin"=0, "depthClampMax"=65535, "disparityMultiplier"=0, "disparityShift(0-127)"=0}  # Depth Table
      w167 = cluster{"meanIntensitySetpoint":u32} {"meanIntensitySetpoint"=800}  # ST_AE_Control
      w171 = T12 {"lambdaCensus"=26.0, "lambdaAD"=2100.0, "ignoreSAD"=0}  # HDAD*
      w170 = T19 {"SLOdiffThreshRed(76)"=300, "SLODiffThreshGreen(77)"=300, "SLODiffThreshBlue(78)"=300}  # ST SLO Threshold
      w172 = T20 {"disableSADColor(68)"=0, "disableRAUColor(69)"=0, "disableSLORightColor(70)"=0, "disableSLOLeftColor(71)"=0, "disableSADNormalize(72)"=0}  # ST Color Control
      w173 = T17 {"rauDiffThreshRed(73)"=600, "rauDiffThreshGreen(74)"=600, "rauDiffThreshBlue(75)"=600}  # ST Rau Threshold
      w174 = T18 {"sloK1Penalty (79)"=44, "sloK2Penalty (80)"=502, "sloK1PenaltyMod1(81)"=23, "sloK2PenaltyMod1(82)"=237, "sloK1PenaltyMod2(83)"=219, "sloK2PenaltyMod2(84)"=113}  # ST SLO Penalty
      w175 = T21 {"plusIncrement (47)"=10, "MinusDecrement (46)"=10, "deepSeaMedianThreshold (48)"=528, "scoreThreshA(49)"=10, "scoreThreshB (50)"=1023, "textureDifferenceThreshold (52)"=0, "textureCountThreshold (51)"=0, "deepSea2ndPeakThresh.(53)"=27, "deepSeaNeighborThresh.(54)"=20, "LRAgreeThreshold (55)"=70}  # depth control
      w176 = T16 {"minWest (60)"=1, "minEast (61)"=1, "minWEsum (62)"=1, "minNorth (63)"=1, "minSouth (64)"=1, "minNSSum(65)"=1, "uStrink (66)"=1, "vShrink (67)"=1}  # ST RAU vector
      w177 = T13 {"rsmBypass (56)"=0, "diffThresh (57)"=7.0, "sloRauDiffThresh(58)"=3.0, "removeThresh(59)"=33}  # ST RSM
    }
    frame "Face2" {
      w179 = cluster{"uDiameter":u32, "vDiameter":u32} {"uDiameter"=9, "vDiameter"=9}  # ST_CensusEnable
      w180 = T15 {"depthUnits, um"=1000, "depthClampMin"=0, "depthClampMax"=65535, "disparityMultiplier"=0, "disparityShift(0-127)"=0}  # Depth Table
      w178 = cluster{"meanIntensitySetpoint":u32} {"meanIntensitySetpoint"=800}  # ST_AE_Control
      w182 = T13 {"rsmBypass (56)"=0, "diffThresh (57)"=1.21875, "sloRauDiffThresh(58)"=0.28125, "removeThresh(59)"=83}  # ST RSM
      w183 = T16 {"minWest (60)"=3, "minEast (61)"=2, "minWEsum (62)"=7, "minNorth (63)"=1, "minSouth (64)"=3, "minNSSum(65)"=6, "uStrink (66)"=4, "vShrink (67)"=0}  # ST RAU vector
      w184 = T17 {"rauDiffThreshRed(73)"=18, "rauDiffThreshGreen(74)"=113, "rauDiffThreshBlue(75)"=586}  # ST Rau Threshold
      w185 = T21 {"plusIncrement (47)"=10, "MinusDecrement (46)"=10, "deepSeaMedianThreshold (48)"=528, "scoreThreshA(49)"=10, "scoreThreshB (50)"=1023, "textureDifferenceThreshold (52)"=0, "textureCountThreshold (51)"=0, "deepSea2ndPeakThresh.(53)"=27, "deepSeaNeighborThresh.(54)"=20, "LRAgreeThreshold (55)"=70}  # depth control
      w186 = T20 {"disableSADColor(68)"=0, "disableRAUColor(69)"=0, "disableSLORightColor(70)"=0, "disableSLOLeftColor(71)"=0, "disableSADNormalize(72)"=0}  # ST Color Control
      w187 = T19 {"SLOdiffThreshRed(76)"=279, "SLODiffThreshGreen(77)"=200, "SLODiffThreshBlue(78)"=8}  # ST SLO Threshold
      w188 = T18 {"sloK1Penalty (79)"=55, "sloK2Penalty (80)"=235, "sloK1PenaltyMod1(81)"=326, "sloK2PenaltyMod1(82)"=506, "sloK1PenaltyMod2(83)"=134, "sloK2PenaltyMod2(84)"=206}  # ST SLO Penalty
    }
    frame "Best Box" {
      w190 = cluster{"uDiameter":u32, "vDiameter":u32} {"uDiameter"=9, "vDiameter"=9}  # ST_CensusEnable
      w191 = T15 {"depthUnits, um"=1000, "depthClampMin"=0, "depthClampMax"=65535, "disparityMultiplier"=0, "disparityShift(0-127)"=0}  # Depth Table
      w189 = cluster{"meanIntensitySetpoint":u32} {"meanIntensitySetpoint"=400}  # ST_AE_Control
      w193 = T13 {"rsmBypass (56)"=0, "diffThresh (57)"=1.21875, "sloRauDiffThresh(58)"=0.28125, "removeThresh(59)"=83}  # ST RSM
      w194 = T16 {"minWest (60)"=3, "minEast (61)"=2, "minWEsum (62)"=7, "minNorth (63)"=1, "minSouth (64)"=3, "minNSSum(65)"=6, "uStrink (66)"=4, "vShrink (67)"=0}  # ST RAU vector
      w195 = T17 {"rauDiffThreshRed(73)"=18, "rauDiffThreshGreen(74)"=113, "rauDiffThreshBlue(75)"=586}  # ST Rau Threshold
      w196 = T21 {"plusIncrement (47)"=10, "MinusDecrement (46)"=10, "deepSeaMedianThreshold (48)"=528, "scoreThreshA(49)"=10, "scoreThreshB (50)"=1023, "textureDifferenceThreshold (52)"=0, "textureCountThreshold (51)"=0, "deepSea2ndPeakThresh.(53)"=27, "deepSeaNeighborThresh.(54)"=20, "LRAgreeThreshold (55)"=70}  # depth control
      w197 = T20 {"disableSADColor(68)"=0, "disableRAUColor(69)"=0, "disableSLORightColor(70)"=0, "disableSLOLeftColor(71)"=0, "disableSADNormalize(72)"=0}  # ST Color Control
      w198 = T19 {"SLOdiffThreshRed(76)"=279, "SLODiffThreshGreen(77)"=200, "SLODiffThreshBlue(78)"=8}  # ST SLO Threshold
      w199 = T18 {"sloK1Penalty (79)"=55, "sloK2Penalty (80)"=235, "sloK1PenaltyMod1(81)"=326, "sloK2PenaltyMod1(82)"=506, "sloK1PenaltyMod2(83)"=134, "sloK2PenaltyMod2(84)"=206}  # ST SLO Penalty
    }
    frame "High Density" {
      n2 = Unbundle By Name(T14 {"depth control"={"plusIncrement"=21, "MinusDecrement"=6, "deepSeaMedianThreshold"=789, "scoreThreshA"=96, "scoreThreshB"=1443, "textureDifferenceThreshold"=2466, "textureCountThreshold"=0, "deepSeaSecondPeakThreshold"=222, "deepSeaNeighborThreshold"=12, "IrAgreeThreshold"=18}, "STColorCorrection output"={"colorCorrection 1"=0.54785156, "colorCorrection 2"=0.32910156, "colorCorrection 3"=0.8222656, "colorCorrection 4"=0.109375, "colorCorrection 5"=-0.40527344, "colorCorrection 6"=-1.5253906, "colorCorrection 7"=0.95703125, "colorCorrection 8"=0.89160156, "colorCorrection 9"=0.7675781, "colorCorrection 10"=-0.4794922, "colorCorrection 11"=0.047851562, "colorCorrection 12"=-0.2705078}, "HDAD"={"lambdaCensus"=15.0, "lambdaAD"=618.0, "ignoreSAD"=0}, "ST RSM"={"rsmBypass"=0, "diffThresh"=1.21875, "sloRauDiffThresh"=0.28125, "removeThresh"=82}, "ST SLO Penalty"={"sloK1Penalty"=55, "sloK2Penalty"=235, "sloK1PenaltyMod1"=326, "sloK2PenaltyMod1"=506, "sloK1PenaltyMod2"=134, "sloK2PenaltyMod2"=206}, "ST SLO Threshold"={"SLOdiffThresholdRed"=279, "SLODiffThresholdGreen"=200, "SLODiffThresholdBlue"=8}, "ST Rau Threshold"={"rauDiffThresholdRed"=18, "rauDiffThresholdGreen"=585, "rauDiffThresholdBlue"=112}, "ST Color Control"={"disableSADColor"=0, "disableRAUColor"=0, "disableSLORightColor"=0, "disableSLOLeftColor"=0, "disableSADNormalize"=0}, "ST RAU vector"={"minWest"=3, "minEast"=2, "minWEsum"=7, "minNorth"=1, "minSouth"=3, "minNSSum"=6, "uStrink"=4, "vShrink"=0}, "Depth Table"={"depthUnits, um"=1000, "depthClampMin"=0, "depthClampMax"=65535, "disparityMultiplier"=0, "disparityShift"=0}, "ST_AE_Control"={"meanIntensitySetpoint"=800}, "ST_CensusEnable"={"uDiameter"=9, "vDiameter"=9}} ("depth settings 2")) -> ("depth control"=w203:T4, "HDAD"=w209:T12, "ST RSM"=w208:T10, "ST SLO Penalty"=w200:T5, "ST SLO Threshold"=w201:T6, "ST Rau Threshold"=w206:T7, "ST Color Control"=w202:T8, "ST RAU vector"=w210:T9, "Depth Table"=w207:T3, "ST_AE_Control"=w204:cluster{"meanIntensitySetpoint":u32}, "ST_CensusEnable"=w205:cluster{"uDiameter":u32, "vDiameter":u32})  [unwired: 1 out]
    }
    frame "Medium Density" {
      n3 = Unbundle By Name(T14 {"depth control"={"plusIncrement"=3, "MinusDecrement"=23, "deepSeaMedianThreshold"=1021, "scoreThreshA"=54, "scoreThreshB"=887, "textureDifferenceThreshold"=0, "textureCountThreshold"=0, "deepSeaSecondPeakThreshold"=600, "deepSeaNeighborThreshold"=97, "IrAgreeThreshold"=19}, "STColorCorrection output"={"colorCorrection 1"=0.4013672, "colorCorrection 2"=0.047851562, "colorCorrection 3"=1.9179688, "colorCorrection 4"=0.54785156, "colorCorrection 5"=-1.5996094, "colorCorrection 6"=-0.48339844, "colorCorrection 7"=1.3095703, "colorCorrection 8"=0.79003906, "colorCorrection 9"=1.9511719, "colorCorrection 10"=-1.9951172, "colorCorrection 11"=0.8769531, "colorCorrection 12"=-0.70410156}, "HDAD"={"lambdaCensus"=26.0, "lambdaAD"=935.0, "ignoreSAD"=0}, "ST RSM"={"rsmBypass"=0, "diffThresh"=1.8125, "sloRauDiffThresh"=1.0, "removeThresh"=81}, "ST SLO Penalty"={"sloK1Penalty"=132, "sloK2Penalty"=342, "sloK1PenaltyMod1"=77, "sloK2PenaltyMod1"=390, "sloK1PenaltyMod2"=234, "sloK2PenaltyMod2"=151}, "ST SLO Threshold"={"SLOdiffThresholdRed"=896, "SLODiffThresholdGreen"=259, "SLODiffThresholdBlue"=16}, "ST Rau Threshold"={"rauDiffThresholdRed"=186, "rauDiffThresholdGreen"=723, "rauDiffThresholdBlue"=14}, "ST Color Control"={"disableSADColor"=0, "disableRAUColor"=0, "disableSLORightColor"=1, "disableSLOLeftColor"=0, "disableSADNormalize"=0}, "ST RAU vector"={"minWest"=5, "minEast"=3, "minWEsum"=11, "minNorth"=1, "minSouth"=3, "minNSSum"=6, "uStrink"=3, "vShrink"=1}, "Depth Table"={"depthUnits, um"=1000, "depthClampMin"=0, "depthClampMax"=65535, "disparityMultiplier"=0, "disparityShift"=0}, "ST_AE_Control"={"meanIntensitySetpoint"=800}, "ST_CensusEnable"={"uDiameter"=9, "vDiameter"=9}} ("depth settings 2")) -> ("depth control"=w216:T4, "HDAD"=w222:T12, "ST RSM"=w221:T10, "ST SLO Penalty"=w213:T5, "ST SLO Threshold"=w214:T6, "ST Rau Threshold"=w219:T7, "ST Color Control"=w215:T8, "ST RAU vector"=w223:T9, "Depth Table"=w220:T3, "ST_AE_Control"=w217:cluster{"meanIntensitySetpoint":u32}, "ST_CensusEnable"=w218:cluster{"uDiameter":u32, "vDiameter":u32})  [unwired: 1 out]
    }
    frame "High Accuracy" {
      n4 = Unbundle By Name(T14 {"depth control"={"plusIncrement"=2, "MinusDecrement"=25, "deepSeaMedianThreshold"=796, "scoreThreshA"=4, "scoreThreshB"=2893, "textureDifferenceThreshold"=1722, "textureCountThreshold"=0, "deepSeaSecondPeakThreshold"=647, "deepSeaNeighborThreshold"=108, "IrAgreeThreshold"=10}, "STColorCorrection output"={"colorCorrection 1"=0.4013672, "colorCorrection 2"=0.047851562, "colorCorrection 3"=1.9179688, "colorCorrection 4"=0.54785156, "colorCorrection 5"=-1.5996094, "colorCorrection 6"=-0.48339844, "colorCorrection 7"=1.3095703, "colorCorrection 8"=0.79003906, "colorCorrection 9"=1.9511719, "colorCorrection 10"=-1.9951172, "colorCorrection 11"=0.8769531, "colorCorrection 12"=-0.70410156}, "HDAD"={"lambdaCensus"=26.0, "lambdaAD"=935.0, "ignoreSAD"=0}, "ST RSM"={"rsmBypass"=0, "diffThresh"=1.65625, "sloRauDiffThresh"=0.71875, "removeThresh"=137}, "ST SLO Penalty"={"sloK1Penalty"=155, "sloK2Penalty"=190, "sloK1PenaltyMod1"=160, "sloK2PenaltyMod1"=507, "sloK1PenaltyMod2"=59, "sloK2PenaltyMod2"=493}, "ST SLO Threshold"={"SLOdiffThresholdRed"=30, "SLODiffThresholdGreen"=15, "SLODiffThresholdBlue"=13}, "ST Rau Threshold"={"rauDiffThresholdRed"=1007, "rauDiffThresholdGreen"=578, "rauDiffThresholdBlue"=803}, "ST Color Control"={"disableSADColor"=0, "disableRAUColor"=0, "disableSLORightColor"=1, "disableSLOLeftColor"=0, "disableSADNormalize"=0}, "ST RAU vector"={"minWest"=2, "minEast"=6, "minWEsum"=12, "minNorth"=3, "minSouth"=2, "minNSSum"=7, "uStrink"=3, "vShrink"=0}, "Depth Table"={"depthUnits, um"=1000, "depthClampMin"=0, "depthClampMax"=65535, "disparityMultiplier"=0, "disparityShift"=0}, "ST_AE_Control"={"meanIntensitySetpoint"=800}, "ST_CensusEnable"={"uDiameter"=9, "vDiameter"=9}} ("depth settings 2")) -> ("depth control"=w228:T4, "HDAD"=w234:T12, "ST RSM"=w233:T10, "ST SLO Penalty"=w225:T5, "ST SLO Threshold"=w226:T6, "ST Rau Threshold"=w231:T7, "ST Color Control"=w227:T8, "ST RAU vector"=w235:T9, "Depth Table"=w232:T3, "ST_AE_Control"=w229:cluster{"meanIntensitySetpoint":u32}, "ST_CensusEnable"=w230:cluster{"uDiameter":u32, "vDiameter":u32})  [unwired: 1 out]
    }
    frame "Hand" {
      n5 = Unbundle By Name(T14 {"depth control"={"plusIncrement"=3, "MinusDecrement"=20, "deepSeaMedianThreshold"=240, "scoreThreshA"=24, "scoreThreshB"=791, "textureDifferenceThreshold"=783, "textureCountThreshold"=0, "deepSeaSecondPeakThreshold"=31, "deepSeaNeighborThreshold"=110, "IrAgreeThreshold"=20}, "STColorCorrection output"={"colorCorrection 1"=0.4013672, "colorCorrection 2"=0.047851562, "colorCorrection 3"=1.9179688, "colorCorrection 4"=0.54785156, "colorCorrection 5"=-1.5996094, "colorCorrection 6"=-0.48339844, "colorCorrection 7"=1.3095703, "colorCorrection 8"=0.79003906, "colorCorrection 9"=1.9511719, "colorCorrection 10"=-1.9951172, "colorCorrection 11"=0.8769531, "colorCorrection 12"=-0.70410156}, "HDAD"={"lambdaCensus"=7.0, "lambdaAD"=1001.0, "ignoreSAD"=0}, "ST RSM"={"rsmBypass"=0, "diffThresh"=3.8125, "sloRauDiffThresh"=0.46875, "removeThresh"=94}, "ST SLO Penalty"={"sloK1Penalty"=63, "sloK2Penalty"=45, "sloK1PenaltyMod1"=14, "sloK2PenaltyMod1"=21, "sloK1PenaltyMod2"=119, "sloK2PenaltyMod2"=12}, "ST SLO Threshold"={"SLOdiffThresholdRed"=618, "SLODiffThresholdGreen"=244, "SLODiffThresholdBlue"=130}, "ST Rau Threshold"={"rauDiffThresholdRed"=141, "rauDiffThresholdGreen"=74, "rauDiffThresholdBlue"=50}, "ST Color Control"={"disableSADColor"=0, "disableRAUColor"=0, "disableSLORightColor"=1, "disableSLOLeftColor"=0, "disableSADNormalize"=0}, "ST RAU vector"={"minWest"=1, "minEast"=3, "minWEsum"=14, "minNorth"=1, "minSouth"=3, "minNSSum"=4, "uStrink"=3, "vShrink"=1}, "Depth Table"={"depthUnits, um"=1000, "depthClampMin"=0, "depthClampMax"=65535, "disparityMultiplier"=0, "disparityShift"=0}, "ST_AE_Control"={"meanIntensitySetpoint"=800}, "ST_CensusEnable"={"uDiameter"=9, "vDiameter"=9}} ("depth settings 2")) -> ("depth control"=w240:T4, "HDAD"=w246:T12, "ST RSM"=w245:T10, "ST SLO Penalty"=w237:T5, "ST SLO Threshold"=w238:T6, "ST Rau Threshold"=w243:T7, "ST Color Control"=w239:T8, "ST RAU vector"=w247:T9, "Depth Table"=w244:T3, "ST_AE_Control"=w241:cluster{"meanIntensitySetpoint":u32}, "ST_CensusEnable"=w242:cluster{"uDiameter":u32, "vDiameter":u32})  [unwired: 1 out]
    }
    frame "Short Range" {
      n6 = Unbundle By Name(T14 {"depth control"={"plusIncrement"=10, "MinusDecrement"=10, "deepSeaMedianThreshold"=528, "scoreThreshA"=10, "scoreThreshB"=1023, "textureDifferenceThreshold"=0, "textureCountThreshold"=0, "deepSeaSecondPeakThreshold"=27, "deepSeaNeighborThreshold"=20, "IrAgreeThreshold"=70}, "STColorCorrection output"={"colorCorrection 1"=0.4013672, "colorCorrection 2"=0.047851562, "colorCorrection 3"=1.9179688, "colorCorrection 4"=0.54785156, "colorCorrection 5"=-1.5996094, "colorCorrection 6"=-0.48339844, "colorCorrection 7"=1.3095703, "colorCorrection 8"=0.79003906, "colorCorrection 9"=1.9511719, "colorCorrection 10"=-1.9951172, "colorCorrection 11"=0.8769531, "colorCorrection 12"=-0.70410156}, "HDAD"={"lambdaCensus"=26.0, "lambdaAD"=935.0, "ignoreSAD"=0}, "ST RSM"={"rsmBypass"=0, "diffThresh"=7.0, "sloRauDiffThresh"=3.0, "removeThresh"=32}, "ST SLO Penalty"={"sloK1Penalty"=44, "sloK2Penalty"=502, "sloK1PenaltyMod1"=23, "sloK2PenaltyMod1"=237, "sloK1PenaltyMod2"=219, "sloK2PenaltyMod2"=113}, "ST SLO Threshold"={"SLOdiffThresholdRed"=300, "SLODiffThresholdGreen"=300, "SLODiffThresholdBlue"=300}, "ST Rau Threshold"={"rauDiffThresholdRed"=599, "rauDiffThresholdGreen"=599, "rauDiffThresholdBlue"=599}, "ST Color Control"={"disableSADColor"=0, "disableRAUColor"=0, "disableSLORightColor"=0, "disableSLOLeftColor"=0, "disableSADNormalize"=0}, "ST RAU vector"={"minWest"=1, "minEast"=1, "minWEsum"=1, "minNorth"=1, "minSouth"=1, "minNSSum"=1, "uStrink"=1, "vShrink"=1}, "Depth Table"={"depthUnits, um"=1000, "depthClampMin"=0, "depthClampMax"=65535, "disparityMultiplier"=0, "disparityShift"=0}, "ST_AE_Control"={"meanIntensitySetpoint"=800}, "ST_CensusEnable"={"uDiameter"=9, "vDiameter"=9}} ("depth settings 2")) -> ("depth control"=w252:T4, "HDAD"=w258:T12, "ST RSM"=w257:T10, "ST SLO Penalty"=w249:T5, "ST SLO Threshold"=w250:T6, "ST Rau Threshold"=w255:T7, "ST Color Control"=w251:T8, "ST RAU vector"=w259:T9, "Depth Table"=w256:T3, "ST_AE_Control"=w253:cluster{"meanIntensitySetpoint":u32}, "ST_CensusEnable"=w254:cluster{"uDiameter":u32, "vDiameter":u32})  [unwired: 1 out]
    }
    frame "Flat wall" {
      # "AndersDepth4"
      n7 = Unbundle By Name(T14 {"depth control"={"plusIncrement"=10, "MinusDecrement"=10, "deepSeaMedianThreshold"=528, "scoreThreshA"=10, "scoreThreshB"=1023, "textureDifferenceThreshold"=0, "textureCountThreshold"=0, "deepSeaSecondPeakThreshold"=27, "deepSeaNeighborThreshold"=20, "IrAgreeThreshold"=70}, "STColorCorrection output"={"colorCorrection 1"=0.4013672, "colorCorrection 2"=0.047851562, "colorCorrection 3"=1.9179688, "colorCorrection 4"=0.54785156, "colorCorrection 5"=-1.5996094, "colorCorrection 6"=-0.48339844, "colorCorrection 7"=1.3095703, "colorCorrection 8"=0.79003906, "colorCorrection 9"=1.9511719, "colorCorrection 10"=-1.9951172, "colorCorrection 11"=0.8769531, "colorCorrection 12"=-0.70410156}, "HDAD"={"lambdaCensus"=26.0, "lambdaAD"=935.0, "ignoreSAD"=0}, "ST RSM"={"rsmBypass"=0, "diffThresh"=7.0, "sloRauDiffThresh"=3.0, "removeThresh"=32}, "ST SLO Penalty"={"sloK1Penalty"=44, "sloK2Penalty"=502, "sloK1PenaltyMod1"=23, "sloK2PenaltyMod1"=237, "sloK1PenaltyMod2"=219, "sloK2PenaltyMod2"=113}, "ST SLO Threshold"={"SLOdiffThresholdRed"=300, "SLODiffThresholdGreen"=300, "SLODiffThresholdBlue"=300}, "ST Rau Threshold"={"rauDiffThresholdRed"=599, "rauDiffThresholdGreen"=599, "rauDiffThresholdBlue"=599}, "ST Color Control"={"disableSADColor"=0, "disableRAUColor"=0, "disableSLORightColor"=0, "disableSLOLeftColor"=0, "disableSADNormalize"=0}, "ST RAU vector"={"minWest"=1, "minEast"=1, "minWEsum"=1, "minNorth"=1, "minSouth"=1, "minNSSum"=1, "uStrink"=1, "vShrink"=1}, "Depth Table"={"depthUnits, um"=1000, "depthClampMin"=0, "depthClampMax"=65535, "disparityMultiplier"=0, "disparityShift"=0}, "ST_AE_Control"={"meanIntensitySetpoint"=800}, "ST_CensusEnable"={"uDiameter"=9, "vDiameter"=9}} ("depth settings 2")) -> ("depth control"=w264:T4, "HDAD"=w270:T12, "ST RSM"=w269:T10, "ST SLO Penalty"=w261:T5, "ST SLO Threshold"=w262:T6, "ST Rau Threshold"=w267:T7, "ST Color Control"=w263:T8, "ST RAU vector"=w271:T9, "Depth Table"=w268:T3, "ST_AE_Control"=w265:cluster{"meanIntensitySetpoint":u32}, "ST_CensusEnable"=w266:cluster{"uDiameter":u32, "vDiameter":u32})  [unwired: 1 out]
    }
    frame "Load .JSON" {
      w273 = cluster{"uDiameter":u32, "vDiameter":u32} {"uDiameter"=9, "vDiameter"=9}  # ST_CensusEnable
      w274 = T15 {"depthUnits, um"=1000, "depthClampMin"=0, "depthClampMax"=65535, "disparityMultiplier"=0, "disparityShift(0-127)"=0}  # Depth Table
      w272 = cluster{"meanIntensitySetpoint":u32} {"meanIntensitySetpoint"=400}  # ST_AE_Control
      n8 = call "File Dialog"("prompt"="Load .JSON file", "pattern (all files)"="*.json") -> ("selected path"=w277:path)  [unwired: 10 in, 3 out]
      n9 = call "rs3_ReadDepthPreference3.vi"("file (use dialog)"=w277) -> ("HDAD 2*"=w280:T12, "ST Color Control 2"=w285:T20, "depth control 2"=w279:T22, "ST RSM 2"=w281:T13, "ST SLO Penalty 2"=w283:T18, "ST SLO Threshold 2"=w284:T19, "ST Rau Threshold 2"=w282:T17, "ST RAU vector 2"=w278:T16)  [unwired: 5 in, 2 out]
    }
    frame "Load .JSON2" {
      n10 = call "File Dialog2"("prompt"="Load .JSON file", "pattern (all files)"="*.json") -> ("selected path"=w291:path)  [unwired: 10 in, 3 out]
      n11 = call "rs3_ReadDepthPreference4.vi"("file (use dialog)"=w291) -> ("HDAD 2*"=w294:T12, "ST_AE_Control"=w288:cluster{"meanIntensitySetpoint":u32}, "ST Color Control 2"=w299:T20, "depth control 2"=w293:T22, "ST RSM 2"=w295:T13, "Depth Table"=w286:T15, "ST SLO Penalty 2"=w297:T18, "ST_CensusEnable"=w287:cluster{"uDiameter":u32, "vDiameter":u32}, "ST SLO Threshold 2"=w298:T19, "ST Rau Threshold 2"=w296:T17, "ST RAU vector 2"=w292:T16)  [unwired: 2 in, 2 out]
    }
  }
  n12 = case shown="\"Custom\"" "Color Presets" {
    tunnel: [w300 T23 {"DS5p- 1"=0.30136988, "colorCorrection 2"=-0.05479452, "colorCorrection 3"=1.9726027, "colorCorrection 4"=0.9041096, "colorCorrection 5"=-0.41095892, "colorCorrection 6"=-1.6438357, "colorCorrection 7"=0.63013697, "colorCorrection 8"=1.7534246, "colorCorrection 9"=1.5068493, "colorCorrection 10"=-2.0, "colorCorrection 11"=1.9726027, "colorCorrection 12"=-1.2876712} ("STColorCorrection") T11 {"colorCorrection 1"=1.339452, "colorCorrection 2"=0.045342464, "colorCorrection 3"=0.80136985, "colorCorrection 4"=0.19479452, "colorCorrection 5"=-1.2150685, "colorCorrection 6"=-0.9254795, "colorCorrection 7"=0.4671233, "colorCorrection 8"=1.3315068, "colorCorrection 9"=1.7899219, "colorCorrection 10"=-1.1794521, "colorCorrection 11"=0.0779452, "colorCorrection 12"=0.049178082} ("STColorCorrection") T11 {"colorCorrection 1"=0.21917808, "colorCorrection 2"=-0.1369863, "colorCorrection 3"=0.79452056, "colorCorrection 4"=0.69452053, "colorCorrection 5"=-0.28095892, "colorCorrection 6"=-1.7138357, "colorCorrection 7"=0.78013694, "colorCorrection 8"=1.4534247, "colorCorrection 9"=0.9368493, "colorCorrection 10"=-1.7, "colorCorrection 11"=1.6836027, "colorCorrection 12"=-0.8076712} ("STColorCorrection") T11 {"colorCorrection 1"=0.5479452, "colorCorrection 2"=0.32876712, "colorCorrection 3"=0.82191783, "colorCorrection 4"=0.10958904, "colorCorrection 5"=-0.4050685, "colorCorrection 6"=-1.5254794, "colorCorrection 7"=0.9571233, "colorCorrection 8"=0.89150685, "colorCorrection 9"=1.189922, "colorCorrection 10"=-0.47945204, "colorCorrection 11"=0.047945205, "colorCorrection 12"=-0.27082193} ("STColorCorrection") T11 {"colorCorrection 1"=0.5479452, "colorCorrection 2"=0.32876712, "colorCorrection 3"=0.37, "colorCorrection 4"=0.11958904, "colorCorrection 5"=-0.044, "colorCorrection 6"=-1.43, "colorCorrection 7"=0.707, "colorCorrection 8"=0.89050686, "colorCorrection 9"=0.766922, "colorCorrection 10"=-0.47945204, "colorCorrection 11"=0.2099452, "colorCorrection 12"=-0.28982192} ("STColorCorrection") w306 T11 {"colorCorrection 1"=-0.1369863, "colorCorrection 2"=1.3424658, "colorCorrection 3"=1.6986301, "colorCorrection 4"=1.7534246, "colorCorrection 5"=-0.8767123, "colorCorrection 6"=-1.9452055, "colorCorrection 7"=1.4520547, "colorCorrection 8"=1.5616438, "colorCorrection 9"=1.479452, "colorCorrection 10"=-2.0, "colorCorrection 11"=1.3972603, "colorCorrection 12"=-0.65753424} ("STColorCorrection") T11 {"colorCorrection 1"=0.30136988, "colorCorrection 2"=-0.05479452, "colorCorrection 3"=1.9726027, "colorCorrection 4"=0.9041096, "colorCorrection 5"=-0.7123288, "colorCorrection 6"=-2.0, "colorCorrection 7"=0.79452056, "colorCorrection 8"=1.99, "colorCorrection 9"=1.3468493, "colorCorrection 10"=-2.0, "colorCorrection 11"=1.8466027, "colorCorrection 12"=-1.3068492} ("STColorCorrection") T11 {"colorCorrection 1"=0.5479452, "colorCorrection 2"=0.32876712, "colorCorrection 3"=0.82191783, "colorCorrection 4"=0.10958904, "colorCorrection 5"=-0.4050685, "colorCorrection 6"=-1.5254794, "colorCorrection 7"=0.9571233, "colorCorrection 8"=0.89150685, "colorCorrection 9"=0.7671233, "colorCorrection 10"=-0.47945204, "colorCorrection 11"=0.047945205, "colorCorrection 12"=-0.27082193} ("STColorCorrection") T11 {"colorCorrection 1"=0.40136987, "colorCorrection 2"=0.047945205, "colorCorrection 3"=1.9178082, "colorCorrection 4"=0.5479452, "colorCorrection 5"=-1.5999494, "colorCorrection 6"=-0.48342466, "colorCorrection 7"=1.3093151, "colorCorrection 8"=0.79, "colorCorrection 9"=1.9508219, "colorCorrection 10"=-1.9952055, "colorCorrection 11"=0.87660265, "colorCorrection 12"=-0.7039726} ("STColorCorrection") w311 w312 w313 w314 w315 T11 {"colorCorrection 1"=0.5479452, "colorCorrection 2"=1.3701172, "colorCorrection 3"=0.65722656, "colorCorrection 4"=0.60253906, "colorCorrection 5"=1.99, "colorCorrection 6"=0.19178082, "colorCorrection 7"=-1.2602739, "colorCorrection 8"=-0.5751953, "colorCorrection 9"=-0.43835616, "colorCorrection 10"=0.24609375, "colorCorrection 11"=-0.7675781, "colorCorrection 12"=1.3154297} ("STColorCorrection") T11 {"colorCorrection 1"=0.12988281, "colorCorrection 2"=0.39941406, "colorCorrection 3"=0.39941406, "colorCorrection 4"=-0.06933594, "colorCorrection 5"=-0.19824219, "colorCorrection 6"=-0.4033203, "colorCorrection 7"=-0.4033203, "colorCorrection 8"=1.0058594, "colorCorrection 9"=0.921875, "colorCorrection 10"=-0.44140625, "colorCorrection 11"=-0.44140625, "colorCorrection 12"=-0.0390625} ("Read color")] -> w3
    tunnel: "STColorCorrection" -> [w300 _ _ _ _ _ _ _ _ _ _ _ _ _ _ _ _ _]
    frame "Custom" {
    }
    frame "RS400 (DS5p)", Default {
    }
    frame "RS400 (DS5p) 2" {
    }
    frame "RS400 (DS5p) 3" {
    }
    frame "RS400 (DS5p) 4" {
    }
    frame "RS400 (DS5p) 5" {
    }
    frame "RS410 (DS5a)" {
      w306 = T11 {"colorCorrection 1"=0.30136988, "colorCorrection 2"=-0.05479452, "colorCorrection 3"=1.9726027, "colorCorrection 4"=0.9041096, "colorCorrection 5"=-0.84931505, "colorCorrection 6"=-1.8082192, "colorCorrection 7"=1.3424658, "colorCorrection 8"=1.7808219, "colorCorrection 9"=1.5068493, "colorCorrection 10"=-2.0, "colorCorrection 11"=1.9726027, "colorCorrection 12"=-1.2876712}  # DS5p
    }
    frame "RS410 (DS5a) 2" {
    }
    frame "DS410 (DS5a) 3" {
    }
    frame "DS410 (DS5a) 4" {
    }
    frame "DS410+IR" {
    }
    frame "DS5LR" {
      w311 = T24 {"Color 0"=0.795, "Color 1"=0.71, "Color 2"=0.493, "Color 3"=0.11, "Color 4"=-0.329, "Color 5"=-1.5902739726027402, "Color 6"=1.1, "Color 7"=1.04, "Color 8"=1.01, "Color 9"=-0.479, "Color 10"=-0.164, "Color 11"=-0.274}  # DS5LR
    }
    frame "DS5LR-2" {
      w312 = T24 {"Color 0"=0.2988, "Color 1"=0.2939, "Color 2"=0.2939, "Color 3"=0.114, "Color 4"=-0.1689, "Color 5"=-0.0849, "Color 6"=-0.0849, "Color 7"=0.5, "Color 8"=0.5, "Color 9"=-0.148, "Color 10"=-0.2109, "Color 11"=-0.081}  # DS5LR1
    }
    frame "DS5LR no pattern" {
      w313 = T24 {"Color 0"=1.9178082191780819, "Color 1"=1.99, "Color 2"=-2.0, "Color 3"=-2.0, "Color 4"=-1.041095890410959, "Color 5"=0.05479452054794498, "Color 6"=-0.2191780821917808, "Color 7"=0.904109589041096, "Color 8"=0.904109589041096, "Color 9"=-0.547945205479452, "Color 10"=-0.13698630136986312, "Color 11"=-0.19178082191780832}  # DS5LR no IR pattern
    }
    frame "RS410 Remove IR" {
      w314 = T24 {"Color 0"=0.4384765625, "Color 1"=1.990234375, "Color 2"=1.990234375, "Color 3"=-2.0, "Color 4"=-1.83984375, "Color 5"=-0.21875, "Color 6"=1.009765625, "Color 7"=1.33984375, "Color 8"=1.73046875, "Color 9"=-1.9951171875, "Color 10"=0.5751953125, "Color 11"=-0.4931640625}  # DS5 no pattern
    }
    frame "RS410 Remove IR 2" {
      w315 = T24 {"Color 0"=0.5205479452054793, "Color 1"=1.99, "Color 2"=1.506849315068493, "Color 3"=-2.0, "Color 4"=-2.0, "Color 5"=-0.08219178082191791, "Color 6"=1.1232876712328768, "Color 7"=1.013698630136986, "Color 8"=1.698630136986301, "Color 9"=-2.0, "Color 10"=0.5753424657534243, "Color 11"=-0.41095890410958913}  # No pattern 3
    }
    frame "DS5micro" {
      (unwired) T11 {"colorCorrection 1"=1.3424658, "colorCorrection 2"=1.369863, "colorCorrection 3"=0.65753424, "colorCorrection 4"=0.60273975, "colorCorrection 5"=1.2876712, "colorCorrection 6"=-0.10958904, "colorCorrection 7"=-0.5753425, "colorCorrection 8"=-0.5753425, "colorCorrection 9"=-1.0410959, "colorCorrection 10"=0.24657534, "colorCorrection 11"=-0.7671233, "colorCorrection 12"=1.3150685} ("STColorCorrection 2")
      (unwired) T11 {"colorCorrection 1"=1.150685, "colorCorrection 2"=1.5068493, "colorCorrection 3"=1.6164384, "colorCorrection 4"=0.08219178, "colorCorrection 5"=1.99, "colorCorrection 6"=-0.7671233, "colorCorrection 7"=-0.82191783, "colorCorrection 8"=-0.60273975, "colorCorrection 9"=0.10958904, "colorCorrection 10"=0.19178082, "colorCorrection 11"=-1.369863, "colorCorrection 12"=1.9452055} ("STColorCorrection")
    }
    frame "D435" {
    }
  }
  n13 = call "rs3 Advanced Set Census Enable Reg3.vi"("error in (no error)"="error in (no error)", "ST_CensusEnableReg"=w9, "device in"="device in") -> ("error out 2"=w76:errorcluster, "error"=w46:u64, "Dev out"=w75:u64)  [unwired: 6 in]
  n14 = call "rs3 Advanced AE setpoint3.vi"("error in (no error)"=w76, "ST_AE_Control"=w7, "device in"=w75) -> ("error out"=w74:errorcluster, "error"=w44:u64, "Dev out"=w73:u64)  [unwired: 6 in]
  n15 = call "rs3 Advanced set depth table control3.vi"("error in (no error)"=w74, "Depth Table"=w5, "device in"=w73) -> ("error out 2"=w72:errorcluster, "error"=w42:u64, "Dev out"=w71:u64)  [unwired: 6 in]
  n16 = call "rs3 Advanced set depth control3.vi"("error in (no error)"=w72, "depth control"=w51, "device in"=w71) -> ("error out"=w70:errorcluster, "error"=w40:u64, "Dev out"=w69:u64)  [unwired: 6 in]
  n17 = call "rs3 Advanced set HDAD3.vi"("error in (no error)"=w70, "HDAD"=w49, "device in"=w69) -> ("error out"=w68:errorcluster, "error"=w39:u64, "Dev out"=w67:u64)  [unwired: 6 in]
  n18 = call "rs3 Advanced set SLO Penalty3.vi"("error in (no error)"=w68, "ST SLO Penalty"=w21, "device in"=w67) -> ("error out"=w66:errorcluster, "error"=w38:u64, "Dev out"=w65:u64)  [unwired: 6 in]
  n19 = call "rs3 Advanced set SLO Threshold3.vi"("error in (no error)"=w66, "ST SLO Threshold"=w18, "device in"=w65) -> ("error out"=w64:errorcluster, "error"=w37:u64, "Dev out"=w63:u64)  [unwired: 6 in]
  n20 = call "rs3 Advanced set RAU control3.vi"("error in (no error)"=w64, "ST RAU vector"=w15, "device in"=w63) -> ("error out"=w62:errorcluster, "error"=w36:u64, "Dev out"=w61:u64)  [unwired: 6 in]
  n21 = call "rs3 Advanced set Rau Threshold3.vi"("error in (no error)"=w62, "ST Rau Threshold"=w16, "device in"=w61) -> ("error out"=w60:errorcluster, "error"=w35:u64, "Dev out"=w59:u64)  [unwired: 6 in]
  n22 = case shown="True" "Set Color Corr" {
    tunnel: w60 -> [w319 w326]
    tunnel: w59 -> [w320 w325]
    tunnel: w3 -> [_ w324]
    tunnel: [w319 w323] -> w58
    tunnel: [w320 w322] -> w57
    tunnel: [u64 0 ("error") w321] -> w33
    frame False {
    }
    frame True {
      n23 = call "rs3 Advanced set color correction3.vi"("error in (no error)"=w326, "STColorCorrection input"=w324, "device in"=w325) -> ("error out"=w323:errorcluster, "error"=w321:u64, "Dev out"=w322:u64)  [unwired: 6 in]
    }
  }
  n24 = case shown="True" TRUE {
    tunnel: w58 -> [w327 w340]
    tunnel: w57 -> [w330 w339]
    tunnel: [w327 w336] -> w56
    tunnel: [w330 w335] -> w55
    tunnel: [u64 0 ("error") w334] -> w34
    tunnel: [u64 0 ("error") w333] -> w32
    tunnel: w13 -> [_ w332]
    tunnel: w11 -> [_ w331]
    frame False {
    }
    frame True {
      n25 = call "rs3 Advanced set Color control3.vi"("error in (no error)"=w340, "ST Color Control"=w331, "device in"=w339) -> ("error out"=w338:errorcluster, "error"=w333:u64, "Dev out"=w337:u64)  [unwired: 6 in]
      n26 = call "rs3 Advanced set RSM control3.vi"("error in (no error)"=w338, "ST RSM"=w332, "device in"=w337) -> ("error out"=w336:errorcluster, "error"=w334:u64, "Dev out"=w335:u64)  [unwired: 6 in]
    }
  }
  "Dev out" <- w55
  "error out" <- w56
  n27 = call "rs3 showError.vi"("error"=w46) -> ("Error summary"=w45:string)  [unwired: 6 in, 4 out]
  n28 = call "rs3 showError.vi"("error"=w44) -> ("Error summary"=w43:string)  [unwired: 6 in, 4 out]
  n29 = call "rs3 showError.vi"("error"=w42) -> ("Error summary"=w41:string)  [unwired: 6 in, 4 out]
  n30 = call "rs3 showError.vi"("error"=w40) -> ("Error summary"=w31:string)  [unwired: 6 in, 4 out]
  n31 = call "rs3 showError.vi"("error"=w39) -> ("Error summary"=w30:string)  [unwired: 6 in, 4 out]
  n32 = call "rs3 showError.vi"("error"=w38) -> ("Error summary"=w29:string)  [unwired: 6 in, 4 out]
  n33 = call "rs3 showError.vi"("error"=w37) -> ("Error summary"=w28:string)  [unwired: 6 in, 4 out]
  n34 = call "rs3 showError.vi"("error"=w36) -> ("Error summary"=w27:string)  [unwired: 6 in, 4 out]
  n35 = call "rs3 showError.vi"("error"=w34) -> ("Error summary"=w48:string)  [unwired: 6 in, 4 out]
  n36 = call "rs3 showError.vi"("error"=w35) -> ("Error summary"=w26:string)  [unwired: 6 in, 4 out]
  n37 = call "rs3 showError.vi"("error"=w33) -> ("Error summary"=w25:string)  [unwired: 6 in, 4 out]
  n38 = call "rs3 showError.vi"("error"=w32) -> ("Error summary"=w23:string)  [unwired: 6 in, 4 out]
  n39 = Concatenate Strings(w45, w24, w43, w24, w41, w24, w31, w24, w30, w24, w29, w24, w28, w24, w27, w24, w48, w24, w26, w24, w25, w24, w23) -> (→"Set advanced error":string)
